vi "Intake_Set.vi"   [LabVIEW 2019]
uses:
  Intake_Globals.vi
  Intake_States.ctl
  Robot Global Data.vi
  <vilib>/Rock Robotics/WPI/DriverStation/WPI_DriverStationRobotMode2.ctl
types:
  T1 = typedef "Intake_States.ctl" = enum16{"Manual_Throttle", "Manual_Single_Speed", "Compliant_Intake", "Command_RunIntake"}
  T2 = typedef "WPI_DriverStationRobotMode2.ctl" = enum16{"Autonomous Disabled", "Autonomous Enabled", "Teleop Disabled", "Teleop Enabled", "Disconnected", "Finish", "Test Disabled", "Test Enabled", "Emergency Stopped"}
  T3 = typedef "Intake_Cluster.ctl" = cluster{"Control_State":T1, "Intake_On":bool, "Intake_Extended":bool, "Intake_Throttle":dbl, "Auto_Notifier":refnum<notifier>, "Parameter_1":dbl, "Parameter_2":dbl, "Step":dbl, "Outtake":bool}
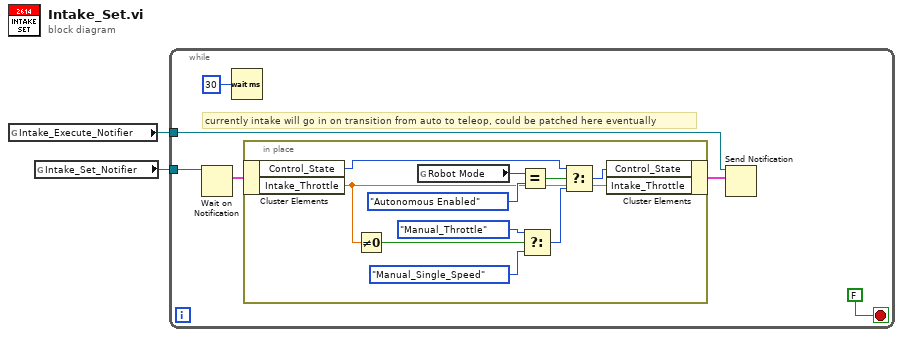
[diagram p0: block diagram]
diagram:
  n1 = global read "Intake_Globals.vi" "Intake_Execute_Notifier"() -> (w1:refnum<notifier>)
  n2 = global read "Intake_Globals.vi" "Intake_Set_Notifier"() -> (w2:refnum<notifier>)
  n3 = while {
    tunnel: w2 -> [w7]
    tunnel: w1 -> [w5]
    stop <- FALSE stop-if-true
    # "currently intake will go in on transition from auto to teleop, could be patched here eventually"
    n4 = Wait on Notification(notifier=w7) -> (notification=w6:T3)  [unwired: 3 in, 3 out]
    n5 = Wait (ms)(milliseconds to wait=u32 30) -> ()  [unwired: 1 out]
    n6 = in-place {
      n7 = in-place-cluster #1(w6) -> ("Control_State"=w14:T1, "Intake_Throttle"=w9:dbl)
      n8 = Not Equal To 0?(x=w9) -> (x != 0?=w11:bool)
      n9 = global read "Robot Global Data.vi" "Robot Mode"() -> (w17:T2)
      n10 = Equal?(x=w17, y=WPI_DriverStationRobotMode2."Autonomous Enabled") -> (x = y?=w15:bool)
      n11 = Select(t=Intake_States."Manual_Throttle" ("Control_State"), s=w11, f=Intake_States."Manual_Single_Speed") -> (s? t:f=w13:T1)
      n12 = Select(t=w14, s=w15, f=w13) -> (s? t:f=w18:T1)
      n13 = in-place-cluster #1("Control_State"=w18, "Intake_Throttle"=w9) -> (w4:T3)
    }
    n14 = Send Notification(notification=w4, notifier=w5) -> ()  [unwired: 1 in, 2 out]
  }
